vi "MFC2.vi"(7 "delay (ms)":u32=500, 11 "Port":refnum<visa-resource-name>="COM1") -> (3 "flow":sgl format="%.3g")   [LabVIEW 2015]
uses:
  MFC_Address.ctl
  Program Files (x86)/National Instruments/LabVIEW 2015/examples/Instrument IO/Serial/support/Serial - Settings.ctl
  <vilib>/Instr/_visa.llb/VISA Configure Serial Port (Instr).vi
panel:
  out "Response":T1
  out "bytes read 2":u32
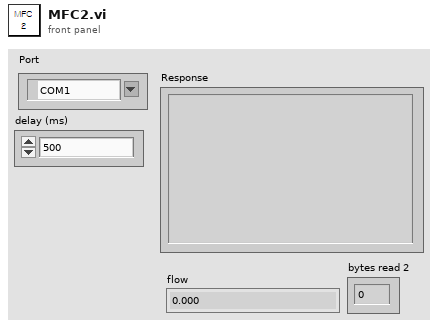
[diagram p1: front panel]
types:
  T1 = typedef "MFC_Address.ctl" = string
  T2 = typedef "Serial - Settings.ctl" = cluster{"baud rate":u32, "data bits":u16, "parity":enum16{"None", "Odd", "Even", "Mark", "Space"}, "stop bits":u16, "flow control":u16}
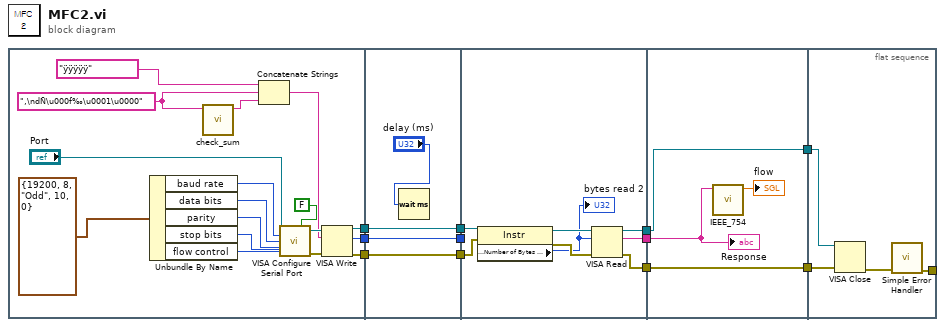
[diagram p0: block diagram]
diagram:
  n1 = flat-sequence {
    tunnel: [w17] -> w11
    tunnel: [w16] -> w10
    tunnel: [w15] -> w9
    tunnel: w11 -> [w31]
    tunnel: w10 -> [w29]
    tunnel: w9 -> [w32]
    tunnel: [w32] -> w8
    tunnel: [w31] -> w7
    tunnel: [w29] -> w3
    tunnel: w8 -> [_]
    tunnel: w7 -> [w37]
    tunnel: [w36] -> w6
    tunnel: [w35] -> w5
    tunnel: w3 -> [w34]
    tunnel: [w33] -> w1
    tunnel: w6 -> [w43]
    tunnel: [w44] -> w4
    tunnel: w5 -> [w44]
    tunnel: [w41] -> w2
    tunnel: w1 -> [w41]
    tunnel: w4 -> [w47]
    tunnel: [w46] -> _
    tunnel: w2 -> [w45]
    frame #0 {
      w12 = "‚\ndÑ\u000f‰\u0001\u0000" ("Command")
      n2 = Unbundle By Name(T2 {"baud rate"=19200, "data bits"=8, "parity"=enum."Odd", "stop bits"=10, "flow control"=0} ("Serial Settings")) -> ("baud rate"=w22:u32, "data bits"=w21:u16, "parity"=w20:enum16{"None", "Odd", "Even", "Mark", "Space"}, "stop bits"=w19:u16, "flow control"=w18:u16)
      n3 = call "check_sum.vi"("command"=w12) -> ("Check Sum"=w14:string)  [unwired: 10 in]
      n4 = Concatenate Strings("ÿÿÿÿÿ" ("문자열"), w12, w14) -> (w24:string)
      n5 = call-poly "VISA Configure Serial Port"("VISA resource name"="Port", "Enable Termination\nChar (T)"=FALSE ("종료문자활성화"), "baud rate (9600)"=w22, "data bits (8)"=w21, "parity (0:none)"=w20, "stop bits (10: 1 bit)"=w19, "flow control (0:none)"=w18) -> ("VISA resource name out"=w26:refnum<visa-resource-name>, "error out"=w27:errorcluster)  [unwired: 2 in, 5 out]
      n6 = VISA Write(VISA resource name=w26, write buffer=w24, error in (no error)=w27) -> (VISA resource name out=w17:refnum<visa-resource-name>, return count=w15:u32, error out=w16:errorcluster)
    }
    frame #1 {
      n7 = Wait (ms)(milliseconds to wait="delay (ms)") -> ()  [unwired: 1 out]
    }
    frame #2 {
      n8 = property class="Instr"(reference=w37, error in=w34) -> (reference out=w40:refnum<visa-resource-name>, error out=w39:errorcluster, "Serial Settings:Number of Bytes at Serial Port"=w38:u32)
      "bytes read 2" <- w38
      n9 = VISA Read(VISA resource name=w40, byte count=w38, error in (no error)=w39) -> (VISA resource name out=w35:refnum<visa-resource-name>, read buffer=w36:string, error out=w33:errorcluster)  [unwired: 1 out]
    }
    frame #3 {
      n10 = call "IEEE_754.vi"("input"=w43) -> ("Return"=→"flow":sgl)  [unwired: 10 in]
      "Response" <- w43
    }
    frame #4 {
      n11 = VISA Close(VISA resource name=w47, error in (no error)=w45) -> (error out=w48:errorcluster)
      n12 = call <vilib>:"Simple Error Handler.vi"("error in (no error)"=w48) -> ("error out"=w46:errorcluster)  [unwired: 1 in, 7 out]
    }
  }
